vi "Remove the sub OD without its main OD.vi"(8 "error in (no error)":errorcluster, 11 "ODs in":T2[](array[typedef]) {"SubNumber" format="%x"; "AccessType" items=["", "ro", "wo", "rw", "const", "rwr", "rww"]; "DataType" items=[""=0, "BOOLEAN"=1, "INTEGER8"=2, "INTEGER16"=3, "INTEGER32"=4, "UNSIGNED8"=5, "UNSIGNED16"=6, "UNSIGNED32"=7, "REAL32"=8, "VISIBLE_STRING"=9, "OCTET_STRING"=10, "UNICODE_STRING"=11, "TIME_OF_DAY"=12, "TIME_DIFFERENCE"=13, "DOMAIN"=15, "INTEGER24"=16, "REAL64"=17, "INTEGER40"=18, "INTEGER48"=19, "INTEGER56"=20, "INTEGER64"=21, "UNSIGNED24"=22, "UNSIGNED40"=24, "UNSIGNED48"=25, "UNSIGNED56"=26, "UNSIGNED64"=27]; "ObjectType" items=[""=10, "NULL"=0, "DOMAIN"=2, "DEFTYPE"=5, "DEFSTRUCT"=6, "VAR"=7, "ARRAY"=8, "RECORD"=9]; "sub-index" format="%x"; "index" format="%x"}) -> (0 "error out":errorcluster, 3 "ODs out":T2[](array[typedef]) {"SubNumber" format="%x"; "AccessType" items=["", "ro", "wo", "rw", "const", "rwr", "rww"]; "DataType" items=[""=0, "BOOLEAN"=1, "INTEGER8"=2, "INTEGER16"=3, "INTEGER32"=4, "UNSIGNED8"=5, "UNSIGNED16"=6, "UNSIGNED32"=7, "REAL32"=8, "VISIBLE_STRING"=9, "OCTET_STRING"=10, "UNICODE_STRING"=11, "TIME_OF_DAY"=12, "TIME_DIFFERENCE"=13, "DOMAIN"=15, "INTEGER24"=16, "REAL64"=17, "INTEGER40"=18, "INTEGER48"=19, "INTEGER56"=20, "INTEGER64"=21, "UNSIGNED24"=22, "UNSIGNED40"=24, "UNSIGNED48"=25, "UNSIGNED56"=26, "UNSIGNED64"=27]; "ObjectType" items=[""=10, "NULL"=0, "DOMAIN"=2, "DEFTYPE"=5, "DEFSTRUCT"=6, "VAR"=7, "ARRAY"=8, "RECORD"=9]; "sub-index" format="%x"; "index" format="%x"})   [LabVIEW 2021, in "CANOpen Addon System Explorer.lvlib"]
uses:
  CANOpen Addon System Explorer.lvlib
  control/OD Entry.ctl
  control/Object Type.ctl
  control/Data Type.ctl
  control/Access Type.ctl
  control/OD Cateory.ctl
  control/Log.ctl
  control/Error Warning Code.ctl
panel:
  in  "ObjectType":T1=7 items=[""=10, "NULL"=0, "DOMAIN"=2, "DEFTYPE"=5, "DEFSTRUCT"=6, "VAR"=7, "ARRAY"=8, "RECORD"=9]
  in  "main OD index":u16
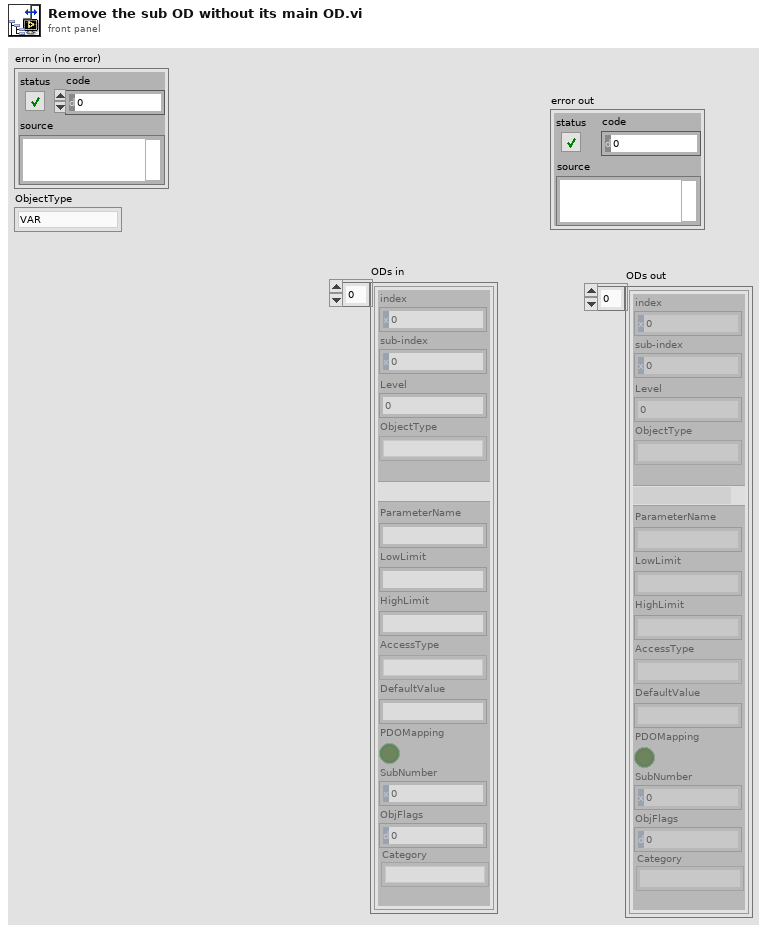
[diagram p1: front panel]
types:
  T1 = typedef "CANOpen Addon System Explorer.lvlib/Object Type.ctl" = u16
  T2 = typedef "CANOpen Addon System Explorer.lvlib/OD Entry.ctl" = cluster{"index":u16, "sub-index":u8, "Level":u8, "ObjectType":T1, "DataType":T3, "ParameterName":string, "LowLimit":string, "HighLimit":string, "AccessType":T4, "DefaultValue":string, "PDOMapping":bool, "SubNumber":u8, "ObjFlags":u32, "Category":T5}
  T3 = typedef "CANOpen Addon System Explorer.lvlib/Data Type.ctl" = u16
  T4 = typedef "CANOpen Addon System Explorer.lvlib/Access Type.ctl" = u16
  T5 = typedef "CANOpen Addon System Explorer.lvlib/OD Cateory.ctl" = enum16{"Mandatory", "Optional", "Manufacturer", ""}
  T6 = typedef "CANOpen Addon System Explorer.lvlib/Log.ctl" = cluster{"Section":string, "Keyword":string, "Value":string, "Error Warning Code":T7}
  T7 = typedef "CANOpen Addon System Explorer.lvlib/Error Warning Code.ctl" = enum16{"SUCCESS", "The data type of OD sub-entry doesn't support the compound and extended type.", "The obect type of the OD sub-entry only supports VAR.", "The multiple data object type can't be changed to single data during the editting mode.", "This OD main-entry can't belong to Manufacture.", "The main-OD or sub-OD had been created.", "The sub-OD doesn't have the main-OD.", "Make suer the object type of main-OD is multiple data.", "It cann't be saved, because of  the value of index is invalid.", "The index is not in our suppprted range.", "Filter the main-OD that address is not in our supported range.", "Don't support object types included NULL and DOMAIN.", "Don't support the Data Types included Boolean, UNICODE_STRING , DOMAIN and reserved.", "The default value can't be parsed. our of range, invalid character", "The sub-index 00 is required.", "Access Type does not support rww and rwr.", "Remove the sub OD that does not have main OD."}
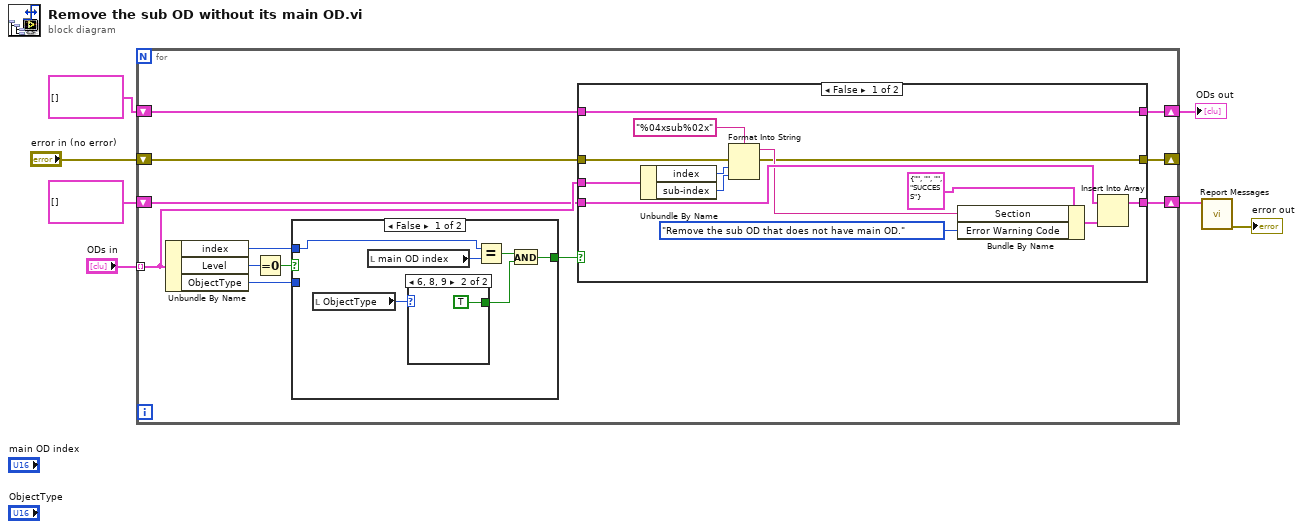
[diagram p0: block diagram]
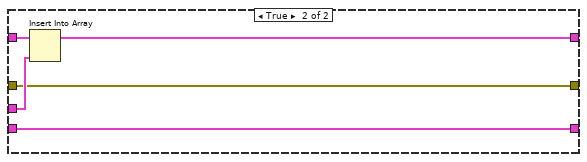
[diagram p2: hidden frame]
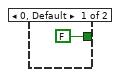
[diagram p3: hidden frame]
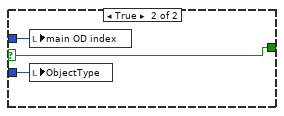
[diagram p4: hidden frame]
diagram:
  n1 = for {
    tunnel: "ODs in" -> [w13] mode=indexing
    shift-right: [w14] -> w5
    shift-left: T2[] [] ("ODs in 2") -> [w15]
    shift-right: [w11] -> w2
    shift-left: T6[] [] ("Logs") -> [w12]
    shift-right: [w9] -> _
    shift-left: "error in (no error)" -> [w10]
    n2 = Unbundle By Name(w13) -> ("index"=w17:u16, "Level"=w19:u8, "ObjectType"=w8:T1)
    n3 = Equal To 0?(x=w19) -> (x = 0?=w18:bool)
    n4 = case shown="False" w18 {
      selector: w18 -> [_ w47]
      tunnel: w17 -> [w42 w48]
      tunnel: [w38 w47] -> w16
      tunnel: w8 -> [_ w46]
      frame False {
        n5 = local read "ObjectType"() -> (w41:T1)
        n6 = local read "main OD index"() -> (w43:u16)
        n7 = case shown="6, 8, 9" w41 {
          tunnel: [FALSE TRUE] -> w39
          frame 0, Default {
          }
          frame 6, 8, 9 {
          }
        }
        n8 = Equal?(x=w42, y=w43) -> (x = y?=w40:bool)
        n9 = And(x=w40, y=w39) -> (x .and. y?=w38:bool)
      }
      frame True {
        n10 = local write "main OD index"(w48) -> ()
        n11 = local write "ObjectType"(w46) -> ()
      }
    }
    n12 = case shown="False" w16 {
      tunnel: w15 -> [w32 w37]
      tunnel: [w32 w36] -> w14
      tunnel: w13 -> [w31 w35]
      tunnel: w12 -> [w30 w34]
      tunnel: [w29 w34] -> w11
      tunnel: w10 -> [w22 w33]
      tunnel: [w21 w33] -> w9
      frame False {
        n13 = Unbundle By Name(w31) -> ("index"=w28:u16, "sub-index"=w27:u8)
        n14 = Format Into String(format string="%04xsub%02x", error in=w22, w28, w27) -> (resulting string=w23:string, error out=w21:errorcluster)  [unwired: 1 in]
        n15 = Bundle By Name(cluster=T6 {"Section"="", "Keyword"="", "Value"="", "Error Warning Code"=enum."SUCCESS"} ("new element/subarray"), "Section"=w23, "Error Warning Code"=Error_Warning_Code."Remove the sub OD that does not have main OD.") -> (w25:T6)
        n16 = Insert Into Array(array=w30, new element=w25) -> (w29:T6[])  [unwired: 1 in]
      }
      frame True {
        n17 = Insert Into Array(array=w37, new element=w35) -> (w36:T2[])  [unwired: 1 in]
      }
    }
  }
  "ODs out" <- w5
  n18 = call "Report Messages.vi"("Logs"=w2) -> ("error out"=→"error out":errorcluster)  [unwired: 9 in, 1 out]
